vi "SCA Sample-Encoder conversion.vi"(6 "Step Window Radius":i16, 7 "Rollover Sample":i8, 9 "Encoder Offset":i16, 10 "Encoder Position":i16, 11 "Desired Sample":u8) -> (1 "Window limit 1":i16, 2 "Within Range?":bool, 3 "Encoder destination":i16, 4 "Window limit 2":i16, 5 "New move (encoder steps)":i16)   [LabVIEW 2016]
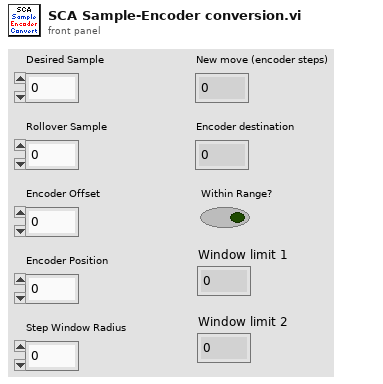
[diagram p1: front panel]
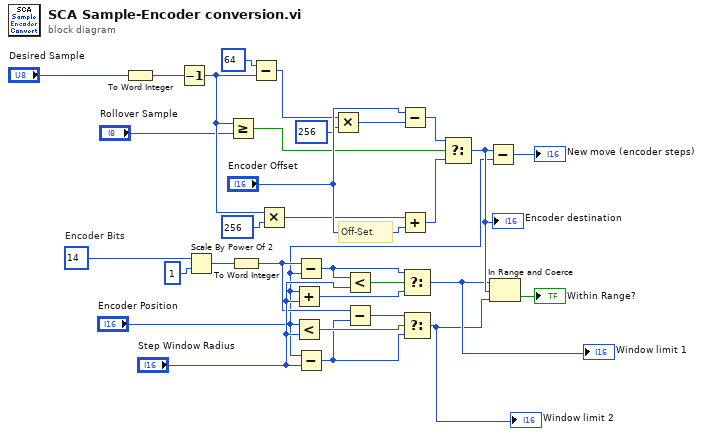
[diagram p0: block diagram]
diagram:
  w27 = i16 14  # Encoder Bits
  # "Off-Set"
  n1 = To Word Integer(number="Desired Sample") -> (16bit integer=w30:i16)
  n2 = Decrement(x=w30) -> (x-1=w25:i16)
  n3 = Scale By Power Of 2(n=w27, x=u32 1) -> (x*2^n=w28:u32)
  n4 = Greater Or Equal?(x=w25, y="Rollover Sample") -> (x >= y?=w21:bool)
  n5 = To Word Integer(number=w28) -> (16bit integer=w2:i16)
  n6 = Subtract(x=i16 64, y=w25) -> (x-y=w19:i16)
  n7 = Multiply(x=w25, y=i16 256) -> (x*y=w13:i16)
  n8 = Add(x="Encoder Position", y="Step Window Radius") -> (x+y=w3:i16)
  n9 = Less?(x="Encoder Position", y="Step Window Radius") -> (x < y?=w9:bool)
  n10 = Subtract(x=w2, y="Encoder Position") -> (x-y=w4:i16)
  n11 = Subtract(x="Encoder Position", y="Step Window Radius") -> (x-y=w6:i16)
  n12 = Multiply(x=w19, y=i16 256) -> (x*y=w20:i16)
  n13 = Less?(x=w4, y="Step Window Radius") -> (x < y?=w5:bool)
  n14 = Subtract(x=w2, y=w6) -> (x-y=w8:i16)
  n15 = Subtract(x="Encoder Offset", y=w20) -> (x-y=w22:i16)
  n16 = Add(x=w13, y="Encoder Offset") -> (x+y=w23:i16)
  n17 = Select(t=w4, s=w5, f=w3) -> (s? t:f=w15:i16)
  "Window limit 1" <- w15
  n18 = Select(t=w8, s=w9, f=w6) -> (s? t:f=w14:i16)
  "Window limit 2" <- w14
  n19 = Select(t=w22, s=w21, f=w23) -> (s? t:f=w24:i16)
  "Encoder destination" <- w24
  n20 = Subtract(x=w24, y="Encoder Position") -> (x-y=→"New move (encoder steps)":i16)
  n21 = In Range and Coerce(upper limit=w15, x=w24, lower limit=w14) -> (In Range?=→"Within Range?":bool)  [unwired: 1 out]
